vi "Rearrange Array 1D Waveforms.vi"(4 "Index Map":i32[](array[numeric]), 6 "Array":waveform(dbl)[](array[waveform])) -> (2 "Rearranged Array":waveform(dbl)[](array[waveform]))   [LabVIEW 2013]
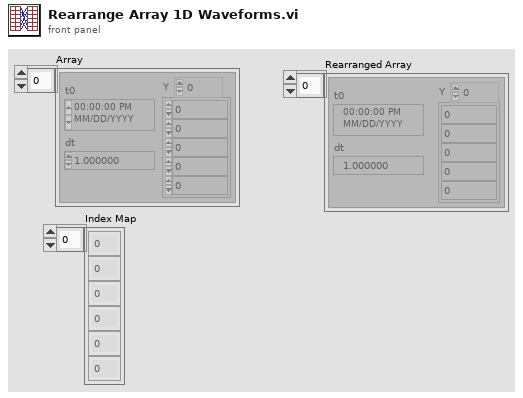
[diagram p1: front panel]
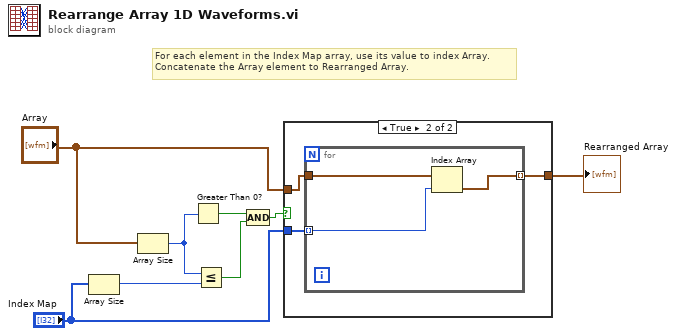
[diagram p0: block diagram]
diagram:
  # "For each element in the Index Map array, use its value to index Array.\nConcatenate the Array element to Rearranged Array."
  n1 = Array Size(array="Index Map") -> (size(s)=w4:i32)
  n2 = Array Size(array="Array") -> (size(s)=w2:i32)
  n3 = Greater Than 0?(x=w2) -> (x > 0?=w6:bool)
  n4 = Less Or Equal?(x=w2, y=w4) -> (x <= y?=w5:bool)
  n5 = Compound Arithmetic op=AND(w6, w5) -> (w7:bool)
  n6 = case shown="True" w7 {
    tunnel: "Index Map" -> [_ w12]
    tunnel: "Array" -> [w9 w10]
    tunnel: [w9 w11] -> w1
    frame False {
    }
    frame True {
      n7 = for {
        tunnel: w12 -> [w13] mode=indexing
        tunnel: w10 -> [w15]
        tunnel: [w14] -> w11 mode=indexing
        n8 = Index Array(array=w15, index=w13) -> (element=w14:waveform(dbl))
      }
    }
  }
  "Rearranged Array" <- w1
